vi "Read Home_.vi"(8 "error in (no error)":errorcluster, 11 "Thorlabs in":refnum<class "Thorlabs.lvclass">) -> (0 "error out":errorcluster, 2 "Home?":bool, 3 "Thorlabs out":refnum<class "Thorlabs.lvclass">)   [LabVIEW 2018]
uses:
  Thorlabs.lvclass
  C:/Projects/LWS_Base/trunk/LabVIEW/PPLs/Axis/Axis.lvlibp/Axis.lvclass
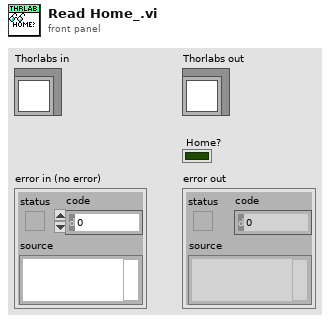
[diagram p1: front panel]
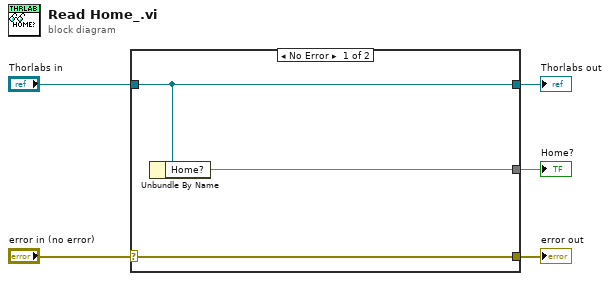
[diagram p0: block diagram]
diagram:
  n1 = case shown="No Error" "error in (no error)" {
    selector: "error in (no error)" -> [w8 w9]
    tunnel: [w8 w9] -> w4
    tunnel: [w7 w10] -> w2
    tunnel: "Thorlabs in" -> [w7 w10]
    tunnel: [w6 _] -> w1
    frame No Error {
      n2 = Unbundle By Name(w7) -> ("Home?"=w6)
    }
    frame Error {
    }
  }
  "error out" <- w4
  "Thorlabs out" <- w2
  "Home?" <- w1
